vi "Configure Stop Trigger [SPT].vi"(7 "Trigger Slope (Positive)":i32(ring) caption="trigger slope (Positive)" items=["Positive", "Negative", "Either"], 8 "error in (no error)":errorcluster, 9 "Trigger Source (None)":string(combo) caption="trigger source (None)", 10 "Channel Name (\"\")":string="CHANNEL1" caption="channel name (\"CHANNEL1\")", 11 "CS++Fgen in":refnum<class "CS++Fgen.lvclass">) -> (0 "error out":errorcluster, 3 "Fgen out":refnum<class "CS++Fgen.lvclass">)   [LabVIEW 2013, in "CS++Fgen.lvlib" / "CS++Fgen.lvclass"]
doc: "This VI configures the properties that control the function generator's stop trigger. These properties are the stop trigger source and slope.\n\nA stop trigger terminates any generation and has the same effect as calling the IviFgen Abort Generation VI.\n\nNote:\n\n(1) This VI is part of the IviFgenStopTrigger [SPT] extension group."
uses:
  CS++Fgen.lvclass
  Core/Classes/CS++ProcessVariables/ProcessVariable/PV.lvclass
  CS++Fgen.lvclass/CS++Fgen.ctl
  Core/Classes/CS++ProcessVariables/PVConnection/PVConnection.lvclass
  Core/Classes/CS++ProcessVariables/ProcessVariable/PV.lvclass/PV.ctl
  Core/Classes/CS++ProcessVariables/ProcessVariable/Write Data.vi
  Core/Classes/CS++ProcessVariables/ProcessVariable/Write Timestamp.vi
  Core/Classes/CS++ProcessVariables/ProcessVariable/Write Quality.vi
  Core/Classes/CS++ProcessVariables/ProcessVariable/Write status.vi
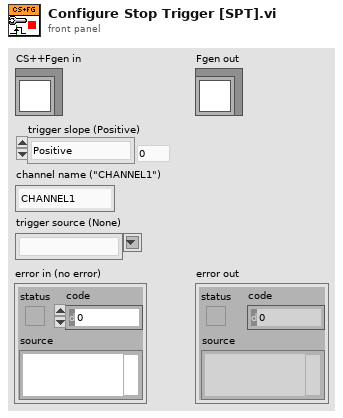
[diagram p1: front panel]
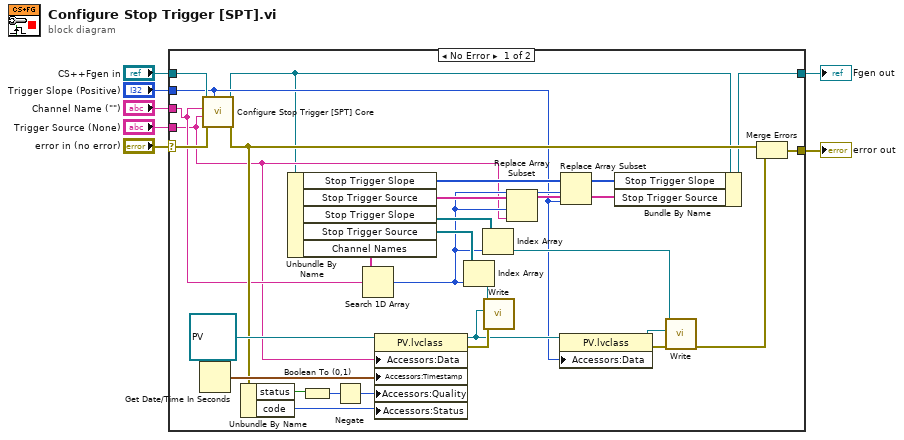
[diagram p0: block diagram]
diagram:
  n1 = case shown="No Error" "error in (no error)" {
    selector: "error in (no error)" -> [w36 w39]
    tunnel: [w8 w39] -> w6
    tunnel: [w9 w38] -> w4
    tunnel: "CS++Fgen in" -> [w37 w38]
    tunnel: "Trigger Slope (Positive)" -> [w11 _]
    tunnel: "Channel Name (\"\")" -> [w13 _]
    tunnel: "Trigger Source (None)" -> [w12 _]
    frame No Error {
      n2 = Get Date/Time In Seconds() -> (seconds since 1Jan1904=w35:timestamp)
      n3 = call-dynamic "Configure Stop Trigger [SPT] Core.vi"("Trigger Slope (Positive)"=w11, "error in (no error)"=w36, "Trigger Source (None)"=w12, "Channel Name (\"\")"=w13, "CS++Fgen in"=w37) -> ("error out"=w14:errorcluster, "Fgen out"=w10:refnum<class "CS++Fgen.lvclass">)  [unwired: 5 in]
      n4 = Unbundle By Name(w14) -> ("status"=w29:bool, "code"=w27:i32)
      n5 = Unbundle By Name(w10) -> ("Stop Trigger Slope"=w23:i32[], "Stop Trigger Source"=w25:string[], "Stop Trigger Slope"=w18:refnum<class "PVConnection.lvclass">[], "Stop Trigger Source"=w31:refnum<class "PVConnection.lvclass">[], "Channel Names"=w32:string[])
      n6 = Boolean To (0,1)(Boolean=w29) -> (0, 1=w28:i16)
      n7 = Negate(x=w28) -> (-x=w26:i16)
      n8 = Search 1D Array(1D array=w32, element=w13) -> (index of element=w17:i32)  [unwired: 1 in]
      n9 = property class="PV.lvclass"(reference=refnum<class "PV.lvclass"> refnum ("PV"), "Accessors:Data"=w12, "Accessors:Timestamp"=w35, "Accessors:Quality"=w26, "Accessors:Status"=w27) -> (reference out=w19:refnum<class "PV.lvclass">, error out=w33:errorcluster)  [unwired: 1 in]
      n10 = Index Array(array=w31, index=w17) -> (element=w30:refnum<class "PVConnection.lvclass">)
      n11 = Index Array(array=w18, index=w17) -> (element=w16:refnum<class "PVConnection.lvclass">)
      n12 = call-dynamic "Write.vi"("error in (no error)"=w33, "PV"=w19, "PVConnection in"=w30) -> ()  [unwired: 7 in, 2 out]
      n13 = Replace Array Subset(array=w25, new element=w12, index=w17) -> (w24:string[])
      n14 = property class="PV.lvclass"(reference=w19, "Accessors:Data"=w11) -> (reference out=w21:refnum<class "PV.lvclass">, error out=w20:errorcluster)  [unwired: 1 in]
      n15 = Replace Array Subset(array=w23, new element=w11, index=w17) -> (w22:i32[])
      n16 = Bundle By Name(cluster=w10, "Stop Trigger Slope"=w22, "Stop Trigger Source"=w24) -> (w9:refnum<class "CS++Fgen.lvclass">)
      n17 = call-dynamic "Write.vi"("error in (no error)"=w20, "PV"=w21, "PVConnection in"=w16) -> ("error out"=w15:errorcluster)  [unwired: 7 in, 1 out]
      n18 = Merge Errors(w14, w15) -> (w8:errorcluster)
    }
    frame Error {
    }
  }
  "error out" <- w6
  "Fgen out" <- w4
